vi "DigitalMonitor.vi"(8 "error in (no error)":errorcluster, 11 "Connection ID":T1) -> (0 "error out":errorcluster, 3 "Connection ID Out":T1)   [LabVIEW 2017, in "GL860_Driver.lvlib"]
uses:
  GL860_Driver.lvlib
  Driver/ConnectionID.ctl
panel:
  out "Digital 20":string
  out "Unit 20":string
  out "Label 20":string
  out "Digital 19":string
  out "Unit 19":string
  out "Label 19":string
  out "Digital 18":string
  out "Unit 18":string
  out "Label 18":string
  out "Digital 17":string
  out "Unit 17":string
  out "Label 17":string
  out "Digital 16":string
  out "Unit 16":string
  out "Label 16":string
  out "Digital 15":string
  out "Unit 15":string
  out "Label 15":string
  out "Digital 14":string
  out "Unit 14":string
  out "Label 14":string
  out "Digital 13":string
  out "Unit 13":string
  out "Label 13":string
  out "Digital 12":string
  out "Unit 12":string
  out "Label 12":string
  out "Digital 11":string
  out "Unit 11":string
  out "Label 11":string
  in  "閉じる":bool
  in  "Sampling":i32(ring)=500 items=["500msec"=500, "1sec"=1000, "2sec"=2000, "5sec"=5000, "10sec"=10000, "20sec"=20000, "30sec"=30000, "1min"=60000, "5min"=300000, "10min"=600000]
  in  "Scrollbar":i32(c297)
  out "Digital 10":string
  out "Unit 10":string
  out "Label 10":string
  out "Digital 9":string
  out "Unit 9":string
  out "Label 9":string
  out "Digital 8":string
  out "Unit 8":string
  out "Label 8":string
  out "Digital 7":string
  out "Unit 7":string
  out "Label 7":string
  out "Digital 6":string
  out "Unit 6":string
  out "Label 6":string
  out "Digital 5":string
  out "Unit 5":string
  out "Label 5":string
  out "Digital 4":string
  out "Unit 4":string
  out "Label 4":string
  out "Digital 3":string
  out "Unit 3":string
  out "Label 3":string
  out "Digital 2":string
  out "Unit 2":string
  out "Label 2":string
  out "Digital 1":string
  out "Unit 1":string
  out "Label 1":string
  # "更新速度"
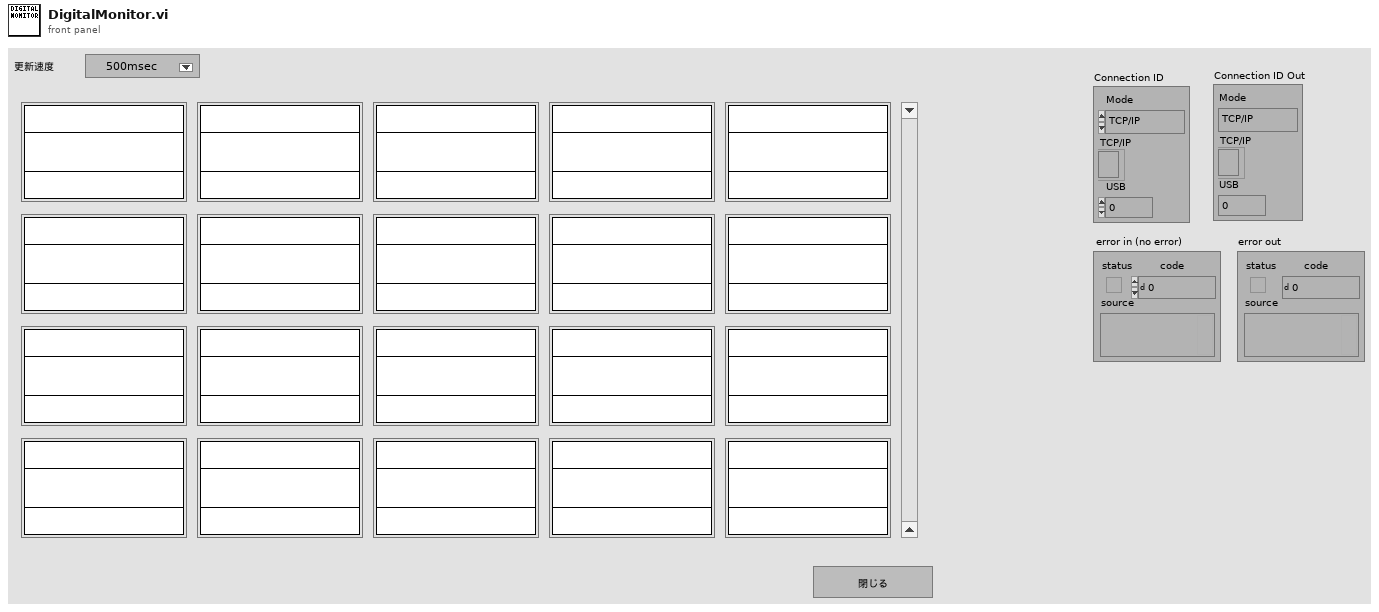
[diagram p1: front panel]
types:
  T1 = typedef "ConnectionID.ctl" = cluster{"Mode":enum16{"TCP/IP", "USB"}, "TCP/IP":refnum<k5>, "USB":i32}
  T2 = cluster{"Meas.Hi":string, "Meas.Lo":string, "Meas.Unit":string, "EU.Hi":string, "EU.Lo":string, "EU.Unit":string}
  T3 = typedef "Amp_Param.ctl" = cluster{"File":refnum<file>[], "Idx":refnum<file>[], "dT":dbl, "Hd":i32, "Rd":i32, "Start":timestamp[], "Trig":timestamp[], "Stop":timestamp[], "FirstPos":timestamp[], "Count":i64[], "Color":u32[], "Label":string[], "INP":string[], "H":dbl[], "L":dbl[], "Fmt":string[], "Unit":string[], "SEL":i32[], "Byte":i32[], "Pos":i32[], "Bit":i32[], "Flg":i32[], "Gain":dbl[], "Offset":dbl[], "CH":i32[], "Opt":cluster{"Mode":i32, "TUNIT":enum16{"CELS", "FAHR"}}, "TYPE":enum16{"GBD", "CSV"}, "Comp":refnum<file>[], "Temp":i32[]}
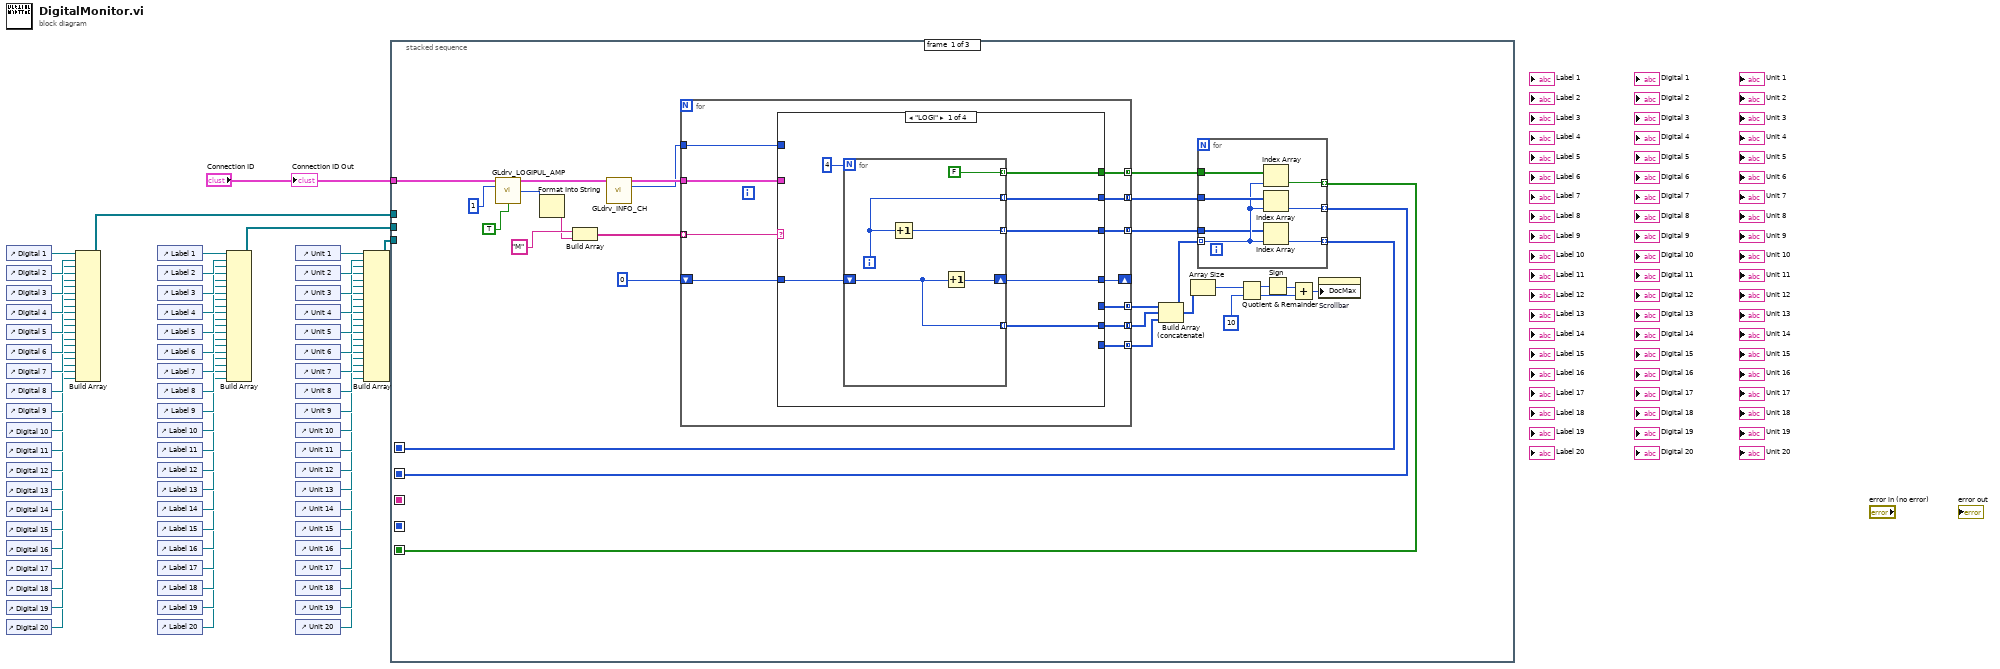
[diagram p0: block diagram]
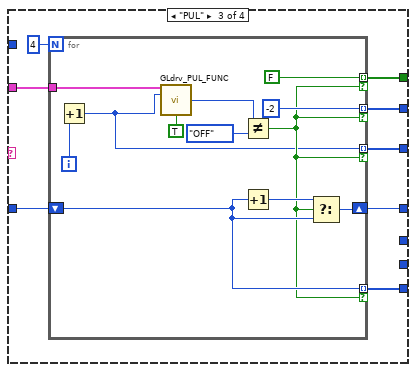
[diagram p3: hidden frame]
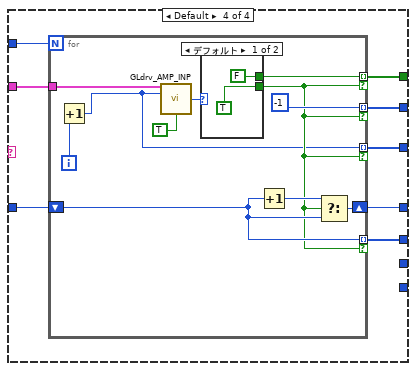
[diagram p4: hidden frame]
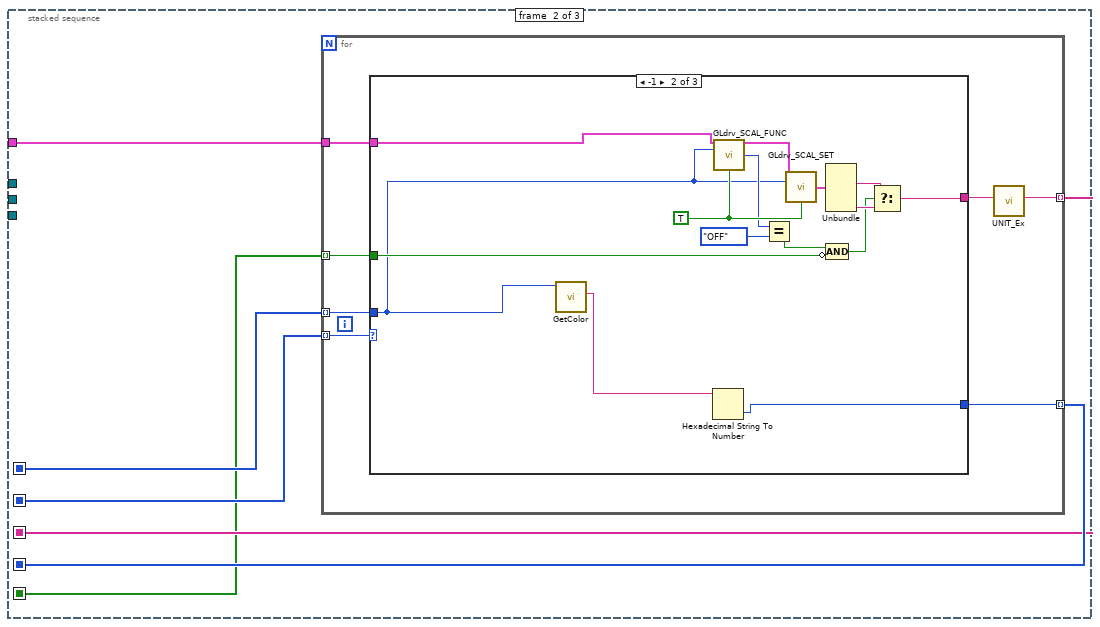
[diagram p6: hidden frame]
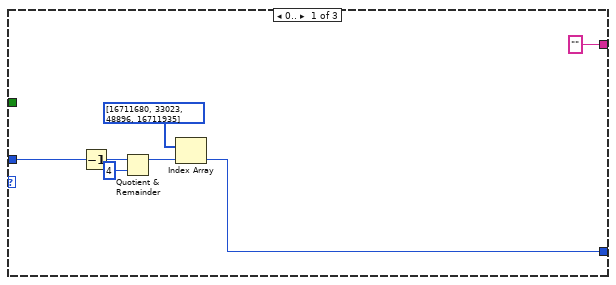
[diagram p7: hidden frame]
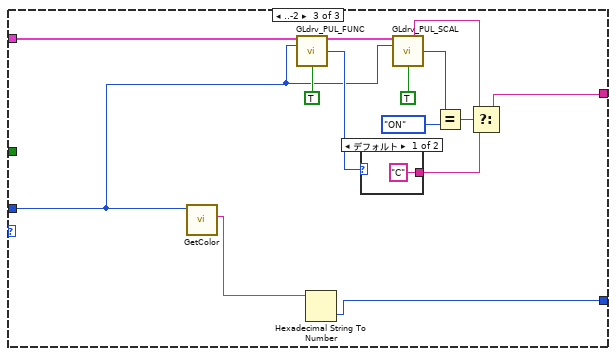
[diagram p8: hidden frame]
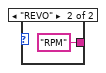
[diagram p9: hidden frame]
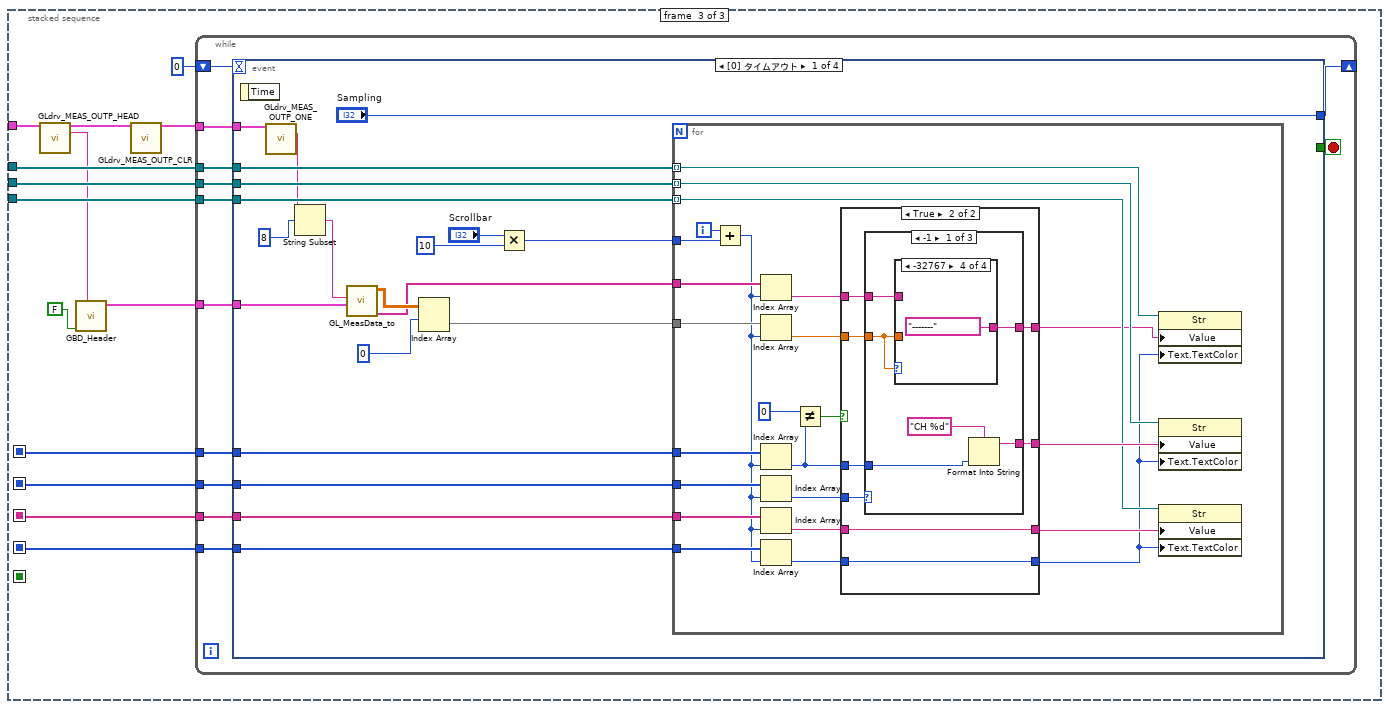
[diagram p10: hidden frame]
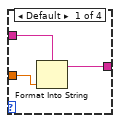
[diagram p12: hidden frame]
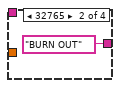
[diagram p13: hidden frame]
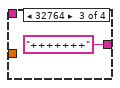
[diagram p14: hidden frame]
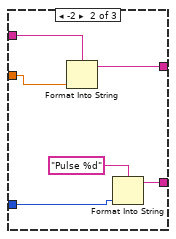
[diagram p15: hidden frame]
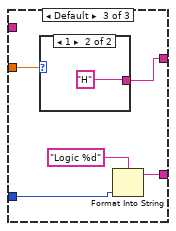
[diagram p16: hidden frame]
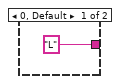
[diagram p17: hidden frame]
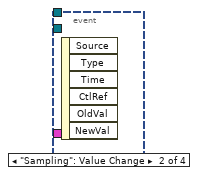
[diagram p18: hidden frame]
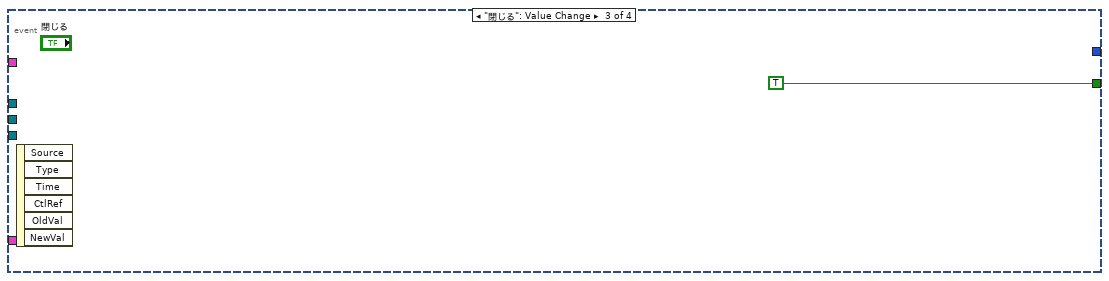
[diagram p19: hidden frame]
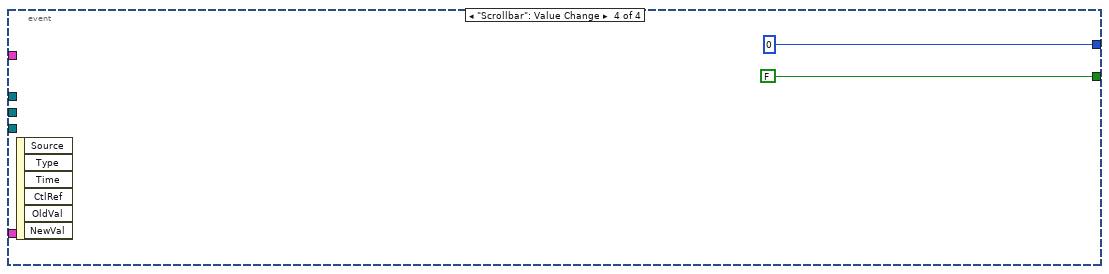
[diagram p20: hidden frame]
diagram:
  n1 = control-ref of="Digital 1"() -> (w44:refnum<vi>)
  n2 = control-ref of="Digital 2"() -> (w43:refnum<vi>)
  n3 = control-ref of="Digital 3"() -> (w42:refnum<vi>)
  n4 = control-ref of="Digital 4"() -> (w41:refnum<vi>)
  n5 = control-ref of="Digital 5"() -> (w40:refnum<vi>)
  n6 = control-ref of="Digital 6"() -> (w39:refnum<vi>)
  n7 = control-ref of="Digital 7"() -> (w38:refnum<vi>)
  n8 = control-ref of="Digital 8"() -> (w37:refnum<vi>)
  n9 = control-ref of="Digital 9"() -> (w36:refnum<vi>)
  n10 = control-ref of="Digital 10"() -> (w35:refnum<vi>)
  n11 = control-ref of="Digital 11"() -> (w34:refnum<vi>)
  n12 = control-ref of="Digital 12"() -> (w33:refnum<vi>)
  n13 = control-ref of="Digital 13"() -> (w32:refnum<vi>)
  n14 = control-ref of="Digital 14"() -> (w31:refnum<vi>)
  n15 = control-ref of="Digital 15"() -> (w30:refnum<vi>)
  n16 = control-ref of="Digital 16"() -> (w29:refnum<vi>)
  n17 = control-ref of="Digital 17"() -> (w28:refnum<vi>)
  n18 = control-ref of="Digital 18"() -> (w27:refnum<vi>)
  n19 = control-ref of="Digital 19"() -> (w26:refnum<vi>)
  n20 = control-ref of="Digital 20"() -> (w25:refnum<vi>)
  n21 = Build Array(w44, w43, w42, w41, w40, w39, w38, w37, w36, w35, w34, w33, w32, w31, w30, w29, w28, w27, w26, w25) -> (w3:refnum<vi>[])
  n22 = control-ref of="Label 1"() -> (w24:refnum<vi>)
  n23 = control-ref of="Label 2"() -> (w23:refnum<vi>)
  n24 = control-ref of="Label 3"() -> (w22:refnum<vi>)
  n25 = control-ref of="Label 4"() -> (w21:refnum<vi>)
  n26 = control-ref of="Label 5"() -> (w20:refnum<vi>)
  n27 = control-ref of="Label 6"() -> (w19:refnum<vi>)
  n28 = control-ref of="Label 7"() -> (w18:refnum<vi>)
  n29 = control-ref of="Label 8"() -> (w17:refnum<vi>)
  n30 = control-ref of="Label 9"() -> (w16:refnum<vi>)
  n31 = control-ref of="Label 10"() -> (w15:refnum<vi>)
  n32 = control-ref of="Label 11"() -> (w14:refnum<vi>)
  n33 = control-ref of="Label 12"() -> (w13:refnum<vi>)
  n34 = control-ref of="Label 13"() -> (w12:refnum<vi>)
  n35 = control-ref of="Label 14"() -> (w11:refnum<vi>)
  n36 = control-ref of="Label 15"() -> (w10:refnum<vi>)
  n37 = control-ref of="Label 16"() -> (w9:refnum<vi>)
  n38 = control-ref of="Label 17"() -> (w8:refnum<vi>)
  n39 = control-ref of="Label 18"() -> (w7:refnum<vi>)
  n40 = control-ref of="Label 19"() -> (w6:refnum<vi>)
  n41 = control-ref of="Label 20"() -> (w5:refnum<vi>)
  n42 = Build Array(w24, w23, w22, w21, w20, w19, w18, w17, w16, w15, w14, w13, w12, w11, w10, w9, w8, w7, w6, w5) -> (w2:refnum<vi>[])
  n43 = control-ref of="Unit 1"() -> (w64:refnum<vi>)
  n44 = control-ref of="Unit 2"() -> (w63:refnum<vi>)
  n45 = control-ref of="Unit 3"() -> (w62:refnum<vi>)
  n46 = control-ref of="Unit 4"() -> (w61:refnum<vi>)
  n47 = control-ref of="Unit 5"() -> (w60:refnum<vi>)
  n48 = control-ref of="Unit 6"() -> (w59:refnum<vi>)
  n49 = control-ref of="Unit 7"() -> (w58:refnum<vi>)
  n50 = control-ref of="Unit 8"() -> (w57:refnum<vi>)
  n51 = control-ref of="Unit 9"() -> (w56:refnum<vi>)
  n52 = control-ref of="Unit 10"() -> (w55:refnum<vi>)
  n53 = control-ref of="Unit 11"() -> (w54:refnum<vi>)
  n54 = control-ref of="Unit 12"() -> (w53:refnum<vi>)
  n55 = control-ref of="Unit 13"() -> (w52:refnum<vi>)
  n56 = control-ref of="Unit 14"() -> (w51:refnum<vi>)
  n57 = control-ref of="Unit 15"() -> (w50:refnum<vi>)
  n58 = control-ref of="Unit 16"() -> (w49:refnum<vi>)
  n59 = control-ref of="Unit 17"() -> (w48:refnum<vi>)
  n60 = control-ref of="Unit 18"() -> (w47:refnum<vi>)
  n61 = control-ref of="Unit 19"() -> (w46:refnum<vi>)
  n62 = control-ref of="Unit 20"() -> (w45:refnum<vi>)
  n63 = Build Array(w64, w63, w62, w61, w60, w59, w58, w57, w56, w55, w54, w53, w52, w51, w50, w49, w48, w47, w46, w45) -> (w4:refnum<vi>[])
  n64 = stacked-sequence {
    seq-local: [_ w167 _] -> [_ _ w223]
    seq-local: [_ w165 _] -> [_ _ w224]
    seq-local: [w85 _ _] -> [_ w169 w222]
    seq-local: [w86 _ _] -> [_ w166 w221]
    seq-local: [w78 _ _] -> [_ w164 _]
    tunnel: w4 -> [_ _ w228]
    tunnel: w3 -> [_ _ w227]
    tunnel: w2 -> [_ _ w226]
    tunnel: "Connection ID" -> [w74 w168 w220]
    frame #0 {
      n65 = call "GLdrv_LOGIPUL_AMP.vi"("Connection ID"=w74, "AMP"=1, "Query(f)"=TRUE) -> ("Connection ID Out"=w70:T1, "Function out"=w76:enum16{"OFF", "LOGI", "PUL"})  [unwired: 10 in, 1 out]
      n66 = Format Into String(w76) -> (resulting string=w75:string)  [unwired: 3 in, 1 out]
      n67 = Build Array("M", w75) -> (w71:string[])
      n68 = call "GLdrv_INFO_CH.vi"("Connection ID"=w70) -> ("Connection ID Out"=w69:T1, "Analog Size out"=w68:i32)  [unwired: 12 in, 1 out]
      n69 = for {
        tunnel: w69 -> [w109]
        tunnel: [w108] -> w87 mode=concatenating
        shift-right: [w106] -> _
        shift-left: 0 -> [w107]
        tunnel: [w105] -> w89 mode=concatenating
        tunnel: [w104] -> w90 mode=concatenating
        tunnel: [w103] -> w88 mode=concatenating
        tunnel: [w102] -> w79 mode=concatenating
        tunnel: w71 -> [w101] mode=indexing
        tunnel: w68 -> [w100]
        tunnel: [w99] -> w67 mode=concatenating
        n70 = case shown="\"LOGI\"" w101 {
          tunnel: w109 -> [_ _ w130 w150]
          tunnel: [w115 _ w128 w149] -> w108
          tunnel: w107 -> [w114 w122 w127 w148]
          tunnel: [w113 w122 w126 w147] -> w106
          tunnel: [w112 _ _ _] -> w105
          tunnel: [_ _ _ w146] -> w104
          tunnel: [_ _ w125 _] -> w103
          tunnel: [w111 _ w124 w145] -> w102
          tunnel: w100 -> [_ _ _ w144]
          tunnel: [w110 _ w123 w143] -> w99
          frame "LOGI" {
            n71 = for {
              N: 4 -> [_]
              tunnel: [w117] -> w110 mode=indexing
              tunnel: [w121] -> w115 mode=indexing
              shift-right: [w119] -> w113
              shift-left: w114 -> [w120]
              tunnel: [w120] -> w112 mode=indexing
              tunnel: [FALSE] -> w111 mode=indexing
              i -> [w121]
              n72 = Increment(x=w121) -> (x+1=w117:i32)
              n73 = Increment(x=w120) -> (x+1=w119:i32)
            }
          }
          frame "OFF" {
          }
          frame "PUL" {
            n74 = for {
              N: 4 -> [_]
              tunnel: w130 -> [w141]
              tunnel: [w131] -> w123 mode=indexing if=w133
              tunnel: [-2] -> w128 mode=indexing if=w133
              shift-right: [w135] -> w126
              shift-left: w127 -> [w134]
              tunnel: [w134] -> w125 mode=indexing if=w133
              tunnel: [FALSE] -> w124 mode=indexing if=w133
              i -> [w142]
              n75 = Increment(x=w142) -> (x+1=w131:i32)
              n76 = call "GLdrv_PUL_FUNC.vi"("Connection ID"=w141, "CH"=w131, "Query(f)"=TRUE) -> ("Function out"=w140:enum16{"OFF", "COUNT", "REVO", "INST"})  [unwired: 10 in, 2 out]
              n77 = Not Equal?(x=w140, y=enum16{"OFF", "COUNT", "REVO", "INST"}."OFF") -> (x != y?=w133:bool)
              n78 = Increment(x=w134) -> (x+1=w136:i32)
              n79 = Select(t=w136, s=w133, f=w134) -> (s? t:f=w135:i32)
            }
          }
          frame Default {
            n80 = for {
              N: w144 -> [_]
              tunnel: w150 -> [w156]
              tunnel: [w151] -> w143 mode=indexing if=w152
              tunnel: [-1] -> w149 mode=indexing if=w152
              shift-right: [w158] -> w147
              shift-left: w148 -> [w157]
              tunnel: [w157] -> w146 mode=indexing if=w152
              tunnel: [w153] -> w145 mode=indexing if=w152
              i -> [w161]
              n81 = Increment(x=w161) -> (x+1=w151:i32)
              n82 = call "GLdrv_AMP_INP.vi"("Connection ID"=w156, "CH"=w151, "Query(f)"=TRUE) -> ("Input out"=w154:enum16{"NONE", "OFF", "DC", "TEMP", "RH"})  [unwired: 2 in, 10 out]
              n83 = case shown="デフォルト" w154 {
                tunnel: [TRUE _] -> w152
                tunnel: [FALSE _] -> w153
                frame Default {
                }
                frame "NONE", "OFF" {
                }
              }
              n84 = Increment(x=w157) -> (x+1=w159:i32)
              n85 = Select(t=w159, s=w152, f=w157) -> (s? t:f=w158:i32)
            }
          }
        }
      }
      n86 = Build Array (concatenate)(w90, w89, w88) -> (w66:i32[])
      n87 = Array Size(array=w66) -> (size(s)=w65:i32)
      n88 = for {
        tunnel: w66 -> [w94] mode=indexing
        tunnel: w87 -> [w98]
        tunnel: [w97] -> w86 mode=indexing
        tunnel: [w96] -> w85 mode=indexing
        tunnel: w79 -> [w95]
        tunnel: [w93] -> w78 mode=indexing
        tunnel: w67 -> [w92]
        n89 = Index Array(array=w95, index=w94) -> (element=w93:bool)
        n90 = Index Array(array=w98, index=w94) -> (element=w97:i32)
        n91 = Index Array(array=w92, index=w94) -> (element=w96:i32)
      }
      n92 = Quotient & Remainder(x=w65, y=10) -> (x-y*floor(x/y)=w83:i32, floor(x/y)=w81:i32)
      n93 = Sign(1:w83) -> (0:w82:i32)
      n94 = Add(x=w82, y=w81) -> (x+y=w80:i32)
      n95 = property on="Scrollbar" class="Scroll （指定）"("DocMax"=w80) -> ()  [unwired: 2 in, 2 out]
    }
    frame #1 {
      n96 = for {
        tunnel: w169 -> [w176] mode=indexing
        tunnel: w168 -> [w175]
        tunnel: [w174] -> w167 mode=indexing
        tunnel: w166 -> [w173] mode=indexing
        tunnel: [w171] -> w165 mode=indexing
        tunnel: w164 -> [w170] mode=indexing
        n97 = case shown="-1" w173 {
          tunnel: w175 -> [_ w187 w202]
          tunnel: [w181 w186 w201] -> w174
          tunnel: w176 -> [w177 w184 w199]
          tunnel: ["" ("Scale In out") w191 w203] -> w172
          tunnel: w170 -> [_ w188 _]
          frame 0.. {
            n98 = Decrement(x=w177) -> (x-1=w178:i32)
            n99 = Quotient & Remainder(x=w178, y=4) -> (x-y*floor(x/y)=w179:i32)  [unwired: 1 out]
            n100 = Index Array(array=u32[] [16711680, 33023, 48896, 16711935], index=w179) -> (element=w181:u32)
          }
          frame -1 {
            w195 = TRUE ("Query(f)")
            n101 = call "GetColor.vi"("CH"=w184) -> ("Strings"=w185:string)  [unwired: 9 in]
            n102 = Hexadecimal String To Number(string=w185) -> (number=w186:u32)  [unwired: 2 in, 1 out]
            n103 = call "GLdrv_SCAL_FUNC.vi"("Connection ID"=w187, "CH"=w184, "Query(f)"=w195) -> ("Connection ID Out"=w192:T1, "Function out"=w193:enum16{"ON", "OFF"})  [unwired: 10 in, 1 out]
            n104 = Equal?(x=w193, y=enum16{"ON", "OFF"}."OFF") -> (x = y?=w198:bool)
            n105 = call "GLdrv_SCAL_SET.vi"("Connection ID"=w192, "CH"=w184, "Query(f)"=w195) -> ("Scale out"=w196:T2)  [unwired: 10 in, 2 out]
            n106 = Unbundle(w196) -> ("Meas.Unit"=w190:string, "EU.Unit"=w197:string)  [unwired: 4 out]
            n107 = Compound Arithmetic op=AND(w198, invert w188) -> (w189:bool)
            n108 = Select(t=w190, s=w189, f=w197) -> (s? t:f=w191:string)
          }
          frame ..-2 {
            n109 = call "GetColor.vi"("CH"=w199) -> ("Strings"=w200:string)  [unwired: 9 in]
            n110 = call "GLdrv_PUL_FUNC.vi"("Connection ID"=w202, "CH"=w199, "Query(f)"=TRUE) -> ("Connection ID Out"=w211:T1, "Function out"=w209:enum16{"OFF", "COUNT", "REVO", "INST"})  [unwired: 10 in, 1 out]
            n111 = Hexadecimal String To Number(string=w200) -> (number=w201:u32)  [unwired: 2 in, 1 out]
            n112 = case shown="デフォルト" w209 {
              tunnel: ["C" ("data out") "RPM" ("data out")] -> w205
              frame Default {
              }
              frame "REVO" {
              }
            }
            n113 = call "GLdrv_PUL_SCAL.vi"("Connection ID"=w211, "CH"=w199, "Query(f)"=TRUE) -> ("Unit out"=w204:string, "Function out"=w208:enum16{"ON", "OFF"})  [unwired: 7 in, 4 out]
            n114 = Equal?(x=w208, y=enum16{"ON", "OFF"}."ON") -> (x = y?=w206:bool)
            n115 = Select(t=w204, s=w206, f=w205) -> (s? t:f=w203:string)
          }
        }
        n116 = call "UNIT_Ex.vi"("In"=w172) -> ("Out"=w171:string)  [unwired: 10 in]
      }
    }
    frame #2 {
      n117 = call "GLdrv_MEAS_OUTP_HEAD.vi"("Connection ID"=w220) -> ("Connection ID Out"=w219:T1, "Header out"=w217:string)  [unwired: 12 in, 1 out]
      n118 = call "GBD_Header.vi"("Head"=w217, "Save?"=FALSE) -> ("Param"=w215:T3)  [unwired: 5 in, 4 out]
      n119 = call "GLdrv_MEAS_OUTP_CLR.vi"("Connection ID"=w219) -> ("Connection ID Out"=w218:T1)  [unwired: 12 in, 2 out]
      n120 = while {
        tunnel: w228 -> [w238]
        tunnel: w227 -> [w237]
        tunnel: w226 -> [w236]
        shift-right: [w239] -> _
        shift-left: 0 ("Sampling") -> [w240]
        tunnel: w218 -> [w234]
        tunnel: w224 -> [w233]
        tunnel: w223 -> [w232]
        tunnel: w222 -> [w231]
        tunnel: w221 -> [w230]
        tunnel: w215 -> [w229]
        stop <- w235 stop-if-true
        n121 = event shown="[0] タイムアウト" {
          selector: _ -> [_ _ _ _]
          dyn-events: _ -> [_ _ _ _]
          timeout: w240 -> [_ _ _ _]
          tunnel: ["Sampling" _ _ 0 ("Sampling")] -> w239
          tunnel: w238 -> [w257 _ _ _]
          tunnel: w237 -> [w258 _ _ _]
          tunnel: w236 -> [w259 _ _ _]
          tunnel: [_ _ TRUE FALSE] -> w235
          tunnel: w234 -> [w248 _ _ _]
          tunnel: w233 -> [w256 _ _ _]
          tunnel: w232 -> [w255 _ _ _]
          tunnel: w231 -> [w251 _ _ _]
          tunnel: w230 -> [w250 _ _ _]
          tunnel: w229 -> [w249 _ _ _]
          event Timeout {
            n122 = event-data() -> ()  [unwired: 1 in, 1 out]
            n123 = call "GLdrv_MEAS_OUTP_ONE.vi"("Connection ID"=w248) -> ("Data out"=w247:string)  [unwired: 12 in, 2 out]
            n124 = String Subset(string=w247, offset (0)=8) -> (substring=w246:string)  [unwired: 1 in]
            n125 = call "GL_MeasData_to.vi"("Ack"=w246, "HEAD"=w249) -> ("Fmt"=w241:string[], "Data"=w245:dbl[][])  [unwired: 4 in, 4 out]
            n126 = Index Array(array=w245, index (row)=0) -> (element=w243:dbl[])  [unwired: 1 in]
            n127 = Multiply(x="Scrollbar", y=10) -> (x*y=w252:i32)
            n128 = for {
              tunnel: w259 -> [w283] mode=indexing
              tunnel: w258 -> [w281] mode=indexing
              tunnel: w257 -> [w280] mode=indexing
              tunnel: w256 -> [w279]
              tunnel: w255 -> [w278]
              tunnel: w252 -> [w277]
              tunnel: w251 -> [w276]
              tunnel: w250 -> [w275]
              tunnel: w243 -> [w273]
              tunnel: w241 -> [w265]
              i -> [w284]
              n129 = Add(x=w284, y=w277) -> (x+y=w264:i32)
              n130 = Index Array(array=w265, index=w264) -> (element=w263:string)
              n131 = Index Array(array=w273, index=w264) -> (element=w266:dbl)
              n132 = Index Array(array=w276, index=w264) -> (element=w272:i32)
              n133 = Index Array(array=w275, index=w264) -> (element=w274:i32)
              n134 = Index Array(array=w279, index=w264) -> (element=w270:string)
              n135 = Index Array(array=w278, index=w264) -> (element=w268:u32)
              n136 = Not Equal?(x=0, y=w272) -> (x != y?=w271:bool)
              n137 = case shown="TRUE" w271 {
                tunnel: [_ w292] -> w282
                tunnel: w274 -> [_ w291]
                tunnel: w272 -> [_ w290]
                tunnel: w270 -> [_ w289]
                tunnel: [_ w289] -> w269
                tunnel: w268 -> [_ w288]
                tunnel: [_ w288] -> w267
                tunnel: w266 -> [_ w285]
                tunnel: w263 -> [_ w286]
                tunnel: [_ w287] -> w262
                frame False {
                }
                frame True {
                  n138 = case shown="-1" w291 {
                    tunnel: [w297 w309 w314] -> w292
                    tunnel: w290 -> [w294 w305 w311]
                    tunnel: [w296 w308 w312] -> w287
                    tunnel: w286 -> [w295 w307 _]
                    tunnel: w285 -> [w293 w306 w313]
                    frame -1 {
                      n139 = case shown="-32767" w293 {
                        tunnel: [w301 "BURN OUT" "+++++++" "-------"] -> w296
                        tunnel: w295 -> [w300 _ _ _]
                        tunnel: w293 -> [w299 _ _ _]
                        frame Default {
                          n140 = Format Into String(format string=w300, w299) -> (resulting string=w301:string)  [unwired: 2 in, 1 out]
                        }
                        frame 32765 {
                        }
                        frame 32764 {
                        }
                        frame -32767 {
                        }
                      }
                      n141 = Format Into String(format string="CH %d", w294) -> (resulting string=w297:string)  [unwired: 2 in, 1 out]
                    }
                    frame -2 {
                      n142 = Format Into String(format string=w307, w306) -> (resulting string=w308:string)  [unwired: 2 in, 1 out]
                      n143 = Format Into String(format string="Pulse %d", w305) -> (resulting string=w309:string)  [unwired: 2 in, 1 out]
                    }
                    frame Default {
                      n144 = case shown="1" w313 {
                        tunnel: ["L" "H"] -> w312
                        frame 0, Default {
                        }
                        frame 1 {
                        }
                      }
                      n145 = Format Into String(format string="Logic %d", w311) -> (resulting string=w314:string)  [unwired: 2 in, 1 out]
                    }
                  }
                }
              }
              n146 = property class="Str"(reference=w281, "Value"=w262, "Text.TextColor"=w267) -> ()  [unwired: 1 in, 2 out]
              n147 = property class="Str"(reference=w283, "Value"=w282, "Text.TextColor"=w267) -> ()  [unwired: 1 in, 2 out]
              n148 = property class="Str"(reference=w280, "Value"=w269, "Text.TextColor"=w267) -> ()  [unwired: 1 in, 2 out]
            }
          }
          event "Sampling": Value Change {
            n149 = event-data() -> ()  [unwired: 1 in, 6 out]
          }
          event "閉じる": Value Change {
            n150 = event-data() -> ()  [unwired: 1 in, 6 out]
          }
          event "Scrollbar": Value Change {
            n151 = event-data() -> ()  [unwired: 1 in, 6 out]
          }
        }
      }
    }
  }
  "Connection ID Out" <- "Connection ID"
